vi "Test SenseHat Reset.vi"() -> ()   [LabVIEW 2020]
uses:
  <vilib>/MakerHub/LINX/Public/Utilities/Open Local.vi
  <vilib>/MakerHub/LINX/LMH-LINX.lvlib
  Classes/SenseHat.Display/RPI.SenseHat.Display.lvclass
panel:
  out "Device Name":string
  out "Error Out":errorcluster
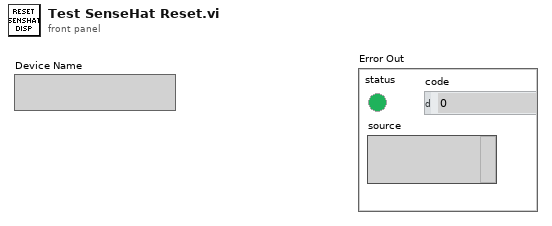
[diagram p1: front panel]
types:
  T1 = typedef "LMH-LINX.lvlib/LINX Ref.ctl" = cluster{"IO":T2, "Interface":T3, "LINX Device Config":T4}
  T2 = typedef "LMH-LINX.lvlib/Platform.ctl" = enum16{"Remote", "Local"}
  T3 = typedef "LMH-LINX.lvlib/Interface.ctl" = enum16{"Serial", "TCP"}
  T4 = typedef "LMH-LINX.lvlib/Device.lvlib/LINX Device Config.ctl" = cluster{"Interface":T3, "COM Port":refnum<visa-resource-name>, "TCP Configuration":T5, "Device Family":u8, "Device ID":u8, "Device Name":string, "TCP Ref":refnum<k5>, "Channels":T6}
  T5 = typedef "LMH-LINX.lvlib/Device.lvlib/TCP Config.ctl" = cluster{"IP Address":string, "Port":u16}
  T6 = typedef "LMH-LINX.lvlib/Channels.ctl" = cluster{"DI":u8[], "DO":u8[], "AI":u8[], "AO":u8[], "PWM":u8[], "QE":u8[], "UART":u8[], "I2C 2":u8[], "SPI":u8[], "CAN":u8[], "Servo":u8[], "AI Ref (V)":dbl, "AI Resolution (Bits)":u8, "AO Ref (V)":dbl, "AO Resolution (Bits)":u8}
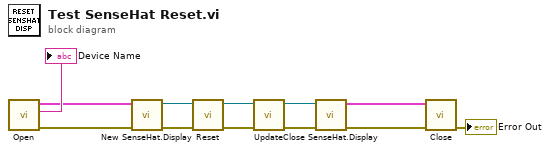
[diagram p0: block diagram]
diagram:
  n1 = call-poly <vilib>:"Open.vi"() -> ("Error Out"=w10:errorcluster, "Device Name"=→"Device Name":string, "LINX Resource"=w3:T1)  [unwired: 9 in]
  n2 = call "New SenseHat.Display.vi"("error in (no error)"=w10, "LINX Resource"=w3) -> ("error out"=w9:errorcluster, "senseHatDisplay out"=w8:refnum<class "RPI.SenseHat.Display.lvclass">)  [unwired: 8 in]
  n3 = call "Reset.vi"("error in (no error)"=w9, "senseHatDisplay in"=w8) -> ("error out"=w2:errorcluster, "senseHatDisplay out"=w1:refnum<class "RPI.SenseHat.Display.lvclass">)  [unwired: 8 in]
  n4 = call "Update.vi"("error in (no error)"=w2, "senseHatDisplay in"=w1) -> ("error out"=w6:errorcluster, "senseHatDisplay out"=w7:refnum<class "RPI.SenseHat.Display.lvclass">)  [unwired: 8 in]
  n5 = call "Close SenseHat.Display.vi"("error in (no error)"=w6, "senseHatDisplay in"=w7) -> ("error out"=w11:errorcluster, "LINX Resource"=w12:T1)  [unwired: 8 in]
  n6 = call <vilib>:"Close.vi"("Error In"=w11, "LINX Resource"=w12) -> ("Error Out"=→"Error Out":errorcluster)  [unwired: 9 in]
